vi "M9003ReciprocalSetup.vi"(8 "Channel (default 1)":u8, 10 "Timeout (0=no timeout)":u32, 11 "HANDLE":i32) -> ()   [LabVIEW 2009]
uses:
  M9003api.dll
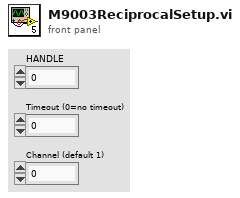
[diagram p1: front panel]
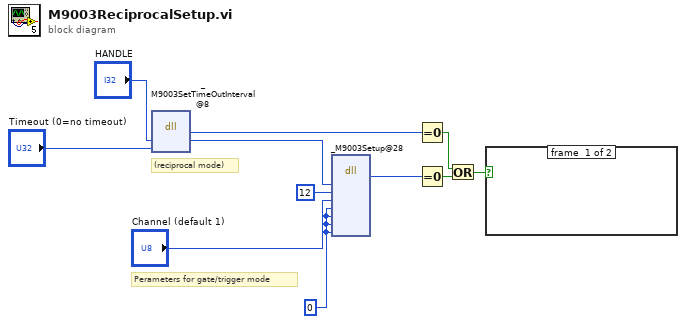
[diagram p0: block diagram]
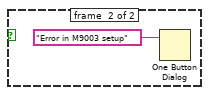
[diagram p2: hidden frame]
diagram:
  w6 = u8 0
  # "Perameters for gate/trigger mode"
  # "(reciprocal mode)"
  n1 = dll-call lib="H:/Mover_2009/Sub_Vis/M9003Commands/M9003api.dll" fn="_M9003SetTimeOutInterval@8" label="M9003SetTimeOutInterval"("Handle"="HANDLE", "Time"="Timeout (0=no timeout)") -> ("return type"=w5:i32, "Handle"=w10:i32)  [unwired: 4 in, 2 out]
  n2 = dll-call lib="H:/Mover_2009/Sub_Vis/M9003Commands/M9003api.dll" fn="_M9003Setup@28" label="M9003Setup"("Handle"=w10, "CountMode"=u8 12, "ChannelEnable"="Channel (default 1)", "TriggerMode"=w6, "GateTime"=w6, "NumberofGate"=w6, "Delimiter"=w6) -> ("return type"=w4:i32)  [unwired: 10 in, 2 out]
  n3 = Equal To 0?(x=w5) -> (x = 0?=w3:bool)
  n4 = Equal To 0?(x=w4) -> (x = 0?=w2:bool)
  n5 = Or(x=w3, y=w2) -> (x .or. y?=w1:bool)
  n6 = case shown="True" w1 {
    frame #0 {
    }
    frame #1 {
      n7 = One Button Dialog(message="Error in M9003 setup") -> ()  [unwired: 1 in, 1 out]
    }
  }
